vi "Stop Core.vi"(10 "final error code":i32, 11 "DIMActor in":refnum<class "DIMActor.lvclass">) -> (3 "DIMActor out":refnum<class "DIMActor.lvclass">)   [LabVIEW 2012, in "DIMActor.lvlib" / "DIMActor.lvclass"]
doc: "Release DIM services, commands and subscribtions."
uses:
  DIMActor.lvclass
  <vilib>/ActorFramework/Actor/Actor.lvclass
  DIMActor.lvclass/DIMActor.ctl
  SVN/LV2009/GPL/lib.lib/DimLVEvent/LVDimInterface/LVDimInterface.lvlib
panel:
  out "Error out":errorcluster
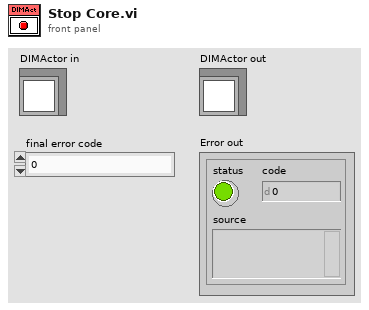
[diagram p1: front panel]
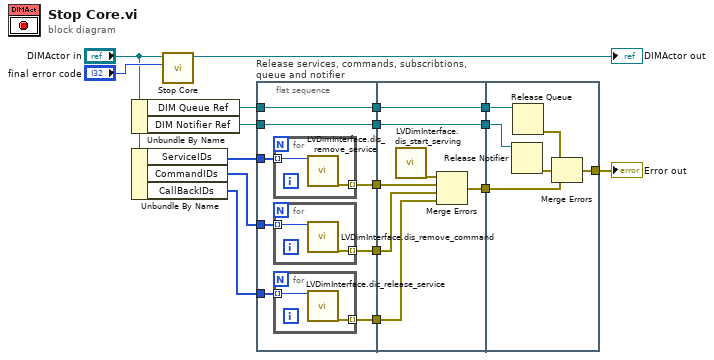
[diagram p0: block diagram]
diagram:
  n1 = Unbundle By Name("DIMActor in") -> ("DIM Queue Ref"=w4:refnum<queue>, "DIM Notifier Ref"=w1:refnum<notifier>)
  n2 = Unbundle By Name("DIMActor in") -> ("ServiceIDs"=w15:i32[], "CommandIDs"=w14:i32[], "CallBackIDs"=w13:i32[])
  n3 = call-parent "Stop Core.vi"("final error code"="final error code", "Actor in"="DIMActor in") -> ("Actor out"=→"DIMActor out":refnum<class "DIMActor.lvclass">)  [unwired: 9 in]
  n4 = flat-sequence "Release services, commands, subscribtions, queue and notifier" {
    tunnel: w15 -> [w25]
    tunnel: w14 -> [w24]
    tunnel: w13 -> [w23]
    tunnel: [w22] -> w12
    tunnel: [w21] -> w11
    tunnel: [w20] -> w10
    tunnel: [w19] -> w5
    tunnel: w4 -> [w19]
    tunnel: [w18] -> w2
    tunnel: w1 -> [w18]
    tunnel: w12 -> [w38]
    tunnel: w11 -> [w37]
    tunnel: w10 -> [w36]
    tunnel: [w35] -> w8
    tunnel: [w34] -> w6
    tunnel: w5 -> [w34]
    tunnel: [w33] -> w3
    tunnel: w2 -> [w33]
    tunnel: [w41] -> w9
    tunnel: w8 -> [w42]
    tunnel: w6 -> [w44]
    tunnel: w3 -> [w43]
    frame #0 {
      n5 = for {
        tunnel: w25 -> [w31] mode=indexing
        tunnel: [w30] -> w22 mode=indexing
        n6 = call "LVDimInterface.dis_remove_service.vi"("my_serviceID"=w31) -> ("error out"=w30:errorcluster)  [unwired: 18 in]
      }
      n7 = for {
        tunnel: w24 -> [w29] mode=indexing
        tunnel: [w28] -> w21 mode=indexing
        n8 = call "LVDimInterface.dis_remove_command.vi"("commandID"=w29) -> ("error out"=w28:errorcluster)  [unwired: 18 in]
      }
      n9 = for {
        tunnel: w23 -> [w27] mode=indexing
        tunnel: [w26] -> w20 mode=indexing
        n10 = call "LVDimInterface.dic_release_service.vi"("callBackID"=w27) -> ("error out"=w26:errorcluster)  [unwired: 18 in]
      }
    }
    frame #1 {
      n11 = call "LVDimInterface.dis_start_serving.vi"() -> ("error out"=w32:errorcluster)  [unwired: 18 in, 1 out]
      n12 = Merge Errors(w32, w38, w37, w36) -> (w35:errorcluster)
    }
    frame #2 {
      n13 = Release Notifier(notifier=w43) -> (error out=w40:errorcluster)  [unwired: 2 in, 2 out]
      n14 = Release Queue(queue=w44) -> (error out=w39:errorcluster)  [unwired: 2 in, 2 out]
      n15 = Merge Errors(w39, w40, w42) -> (w41:errorcluster)
    }
  }
  "Error out" <- w9
